vi "Format Field Display.vi"(10 "size":i32=40, 11 "strings":string[](array[string])) -> (3 "String":string)   [LabVIEW 2011]
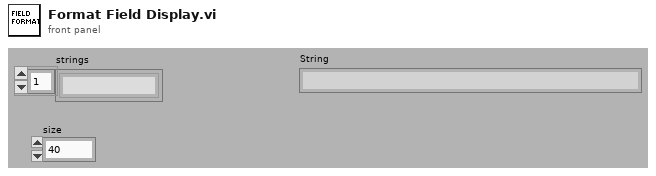
[diagram p1: front panel]
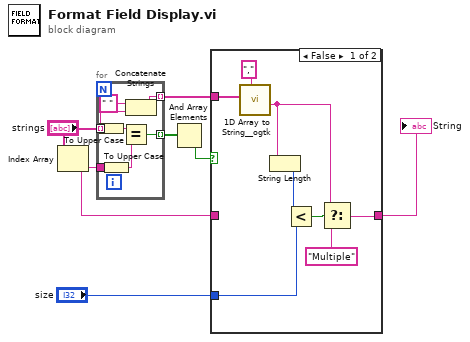
[diagram p0: block diagram]
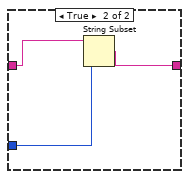
[diagram p2: hidden frame]
diagram:
  n1 = Index Array(array="strings") -> (element=w5:string)  [unwired: 1 in]
  n2 = for {
    tunnel: "strings" -> [w10] mode=indexing
    tunnel: w5 -> [w14]
    tunnel: [w13] -> w7 mode=indexing
    tunnel: [w9] -> w1 mode=indexing
    n3 = To Upper Case(1:w10) -> (0:w12:string)
    n4 = To Upper Case(1:w14) -> (0:w11:string)
    n5 = Equal?(x=w12, y=w11) -> (x = y?=w13:bool)
    n6 = Concatenate Strings(" " ("string"), w10) -> (w9:string)
  }
  n7 = And Array Elements(Boolean array=w7) -> (logical AND=w6:bool)
  n8 = case shown="False" w6 {
    tunnel: w5 -> [_ w25]
    tunnel: [w19 w24] -> w4
    tunnel: "size" -> [w21 w23]
    tunnel: w1 -> [w17 _]
    frame False {
      n9 = call "1D Array to String__ogtk.vi"("delimiter (Tab)"=",", "Array of Strings"=w17) -> ("delimited string"=w15:string)  [unwired: 9 in]
      n10 = String Length(string=w15) -> (length=w22:i32)
      n11 = Less?(x=w22, y=w21) -> (x < y?=w20:bool)
      n12 = Select(t=w15, s=w20, f="Multiple") -> (s? t:f=w19:string)
    }
    frame True {
      n13 = String Subset(string=w25, length (rest)=w23) -> (substring=w24:string)  [unwired: 1 out]
    }
  }
  "String" <- w4
